vi "lab5_KD.vi"(0 "a":dbl, 1 "b":dbl, 2 "Array":dbl[][](array[numeric]), 3 "шаг по времени":dbl, 4 "конец по времени":dbl) -> (5 "Array out":dbl[](array[numeric]))   [LabVIEW 2018]
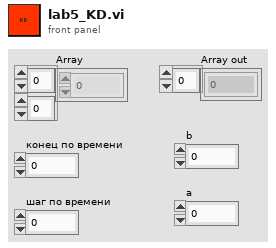
[diagram p1: front panel]
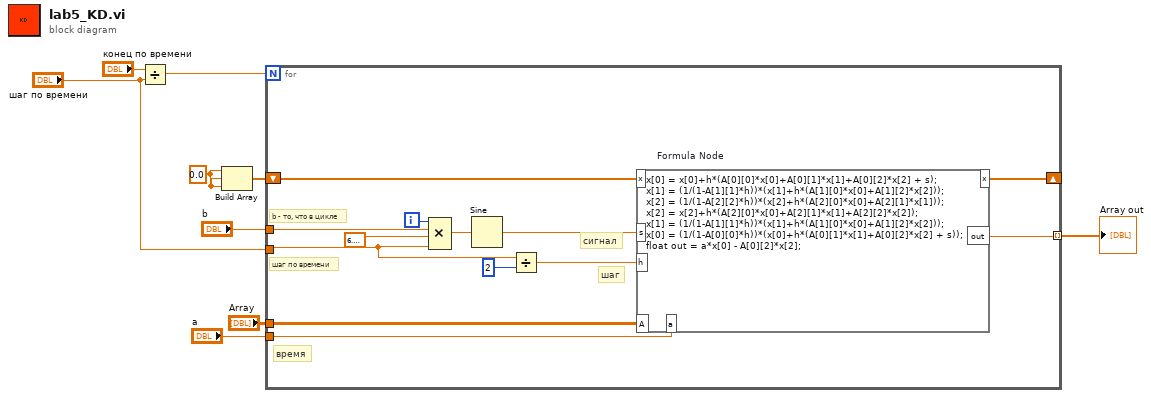
[diagram p0: block diagram]
diagram:
  w3 = 0.0
  n1 = Divide(x="конец по времени", y="шаг по времени") -> (x/y=w4:dbl)
  n2 = Build Array(w3, w3, w3) -> (w2:dbl[])
  n3 = for {
    N: w4 -> [_]
    tunnel: "b" -> [w21]
    tunnel: "шаг по времени" -> [w12]
    tunnel: [w17] -> w7 mode=indexing
    shift-right: [w18] -> _
    shift-left: w2 -> [w19]
    tunnel: "a" -> [w14]
    tunnel: "Array" -> [w13]
    i -> [w15]
    # "шаг по времени"
    # "b - то, что в цикле"
    # "время"
    # "шаг"
    # "сигнал"
    n4 = Compound Arithmetic op=MULTIPLY(6.283185307179586, w21, w15, w12) -> (w20:dbl)
    n5 = Sine(x=w20) -> (sin(x)=w16:dbl)
    n6 = Divide(x=w12, y=2) -> (x/y=w10:dbl)
    n7 = formula code="x[0] = x[0]+h*(A[0][0]*x[0]+A[0][1]*x[1]+A[0][2]*x[2] + s);\nx[1] = (1/(1-A[1][1]*h))*(x[1]+h*(A[1][0]*x[0]+A[1][2]*x[2]));\nx[2] = (1/(1-A[2][2]*h))*(x[2]+h*(A[2][0]*x[0]+A[2][1]*x[1]));\nx[2] = x[2]+h*(A[2][0]*x[0]+A[2][1]*x[1]+A[2][2]*x[2]);\nx[1] = (1/(1-A[1][1]*h))*(x[1]+h*(A[1][0]*x[0]+A[1][2]*x[2]));\nx[0] = (1/(1-A[0][0]*h))*(x[0]+h*(A[0][1]*x[1]+A[0][2]*x[2] + s));\nfloat out = a*x[0] - A[0][2]*x[2];"("x"=w19, "s"=w16, "h"=w10, "A"=w13, "a"=w14) -> ("x"=w18:dbl[], "out"=w17:dbl)
  }
  "Array out" <- w7
